vi "DevTests_UnitCircle.vi"(0 "Quality":i32) -> (1 "Circle":T1[](array[typedef]), 2 "Order":i32[](array[numeric]))   [LabVIEW 2024]
uses:
  SDL3/Rect/FPoint--cluster.ctl
  SDL3/Rect/Rect.lvlib
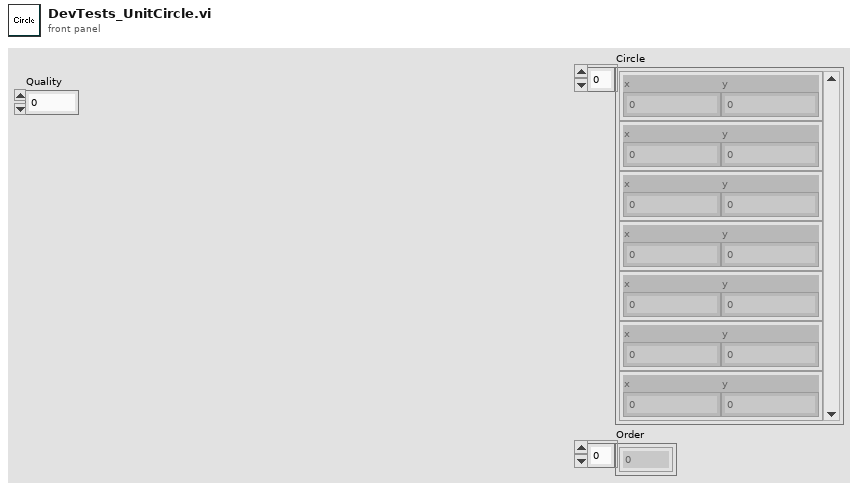
[diagram p1: front panel]
types:
  T1 = typedef "SDL3.lvlib/Rect.lvlib/FPoint--cluster.ctl" = cluster{"x":sgl, "y":sgl}
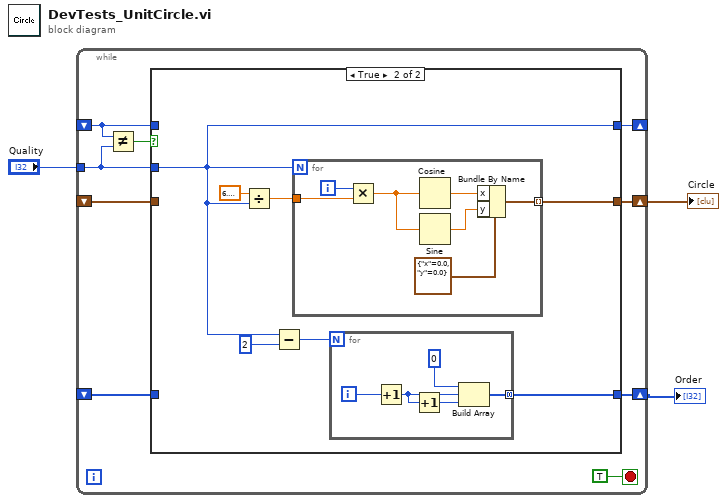
[diagram p0: block diagram]
diagram:
  n1 = while {
    tunnel: "Quality" -> [w9]
    shift-right: [w11] -> w2
    shift-left: _ -> [w10]
    shift-right: [w8] -> _
    shift-left: _ -> [w6]
    shift-right: [w5] -> w1
    shift-left: _ -> [w4]
    stop <- TRUE stop-if-true
    n2 = Not Equal?(x=w6, y=w9) -> (x != y?=w7:bool)
    n3 = case shown="True" w7 {
      tunnel: [w15 w22] -> w11
      tunnel: w10 -> [w15 _]
      tunnel: w9 -> [_ w17]
      tunnel: [w14 w17] -> w8
      tunnel: w6 -> [w14 _]
      tunnel: [w13 w16] -> w5
      tunnel: w4 -> [w13 _]
      frame False {
      }
      frame True {
        n4 = Divide(x=6.283185307179586, y=w17) -> (x/y=w21:dbl)
        n5 = Subtract(x=w17, y=2) -> (x-y=w19:i32)
        n6 = for {
          N: w17 -> [_]
          tunnel: w21 -> [w32]
          tunnel: [w28] -> w22 mode=indexing
          i -> [w33]
          n7 = Multiply(x=w33, y=w32) -> (x*y=w34:dbl)
          n8 = Cosine(x=w34) -> (cos(x)=w30:dbl)
          n9 = Sine(x=w34) -> (sin(x)=w29:dbl)
          n10 = Bundle By Name(cluster=T1 {"x"=0.0, "y"=0.0} ("FPoint"), "x"=w30, "y"=w29) -> (w28:T1)
        }
        n11 = for {
          N: w19 -> [_]
          tunnel: [w23] -> w16 mode=concatenating
          i -> [w27]
          n12 = Increment(x=w27) -> (x+1=w26:i32)
          n13 = Increment(x=w26) -> (x+1=w25:i32)
          n14 = Build Array(0 ("element"), w26, w25) -> (w23:i32[])
        }
      }
    }
  }
  "Circle" <- w2
  "Order" <- w1
